vi "drive_calc.vi"(11 "Drive_inputs":T2) -> (3 "Drive_Outputs":T1)   [LabVIEW 2013]
uses:
  drive_inputs.ctl
  drive_outputs.ctl
panel:
  in  "Drive_Outputs 2":T1
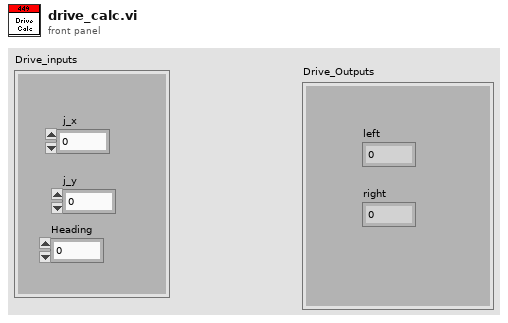
[diagram p1: front panel]
types:
  T1 = typedef "drive_outputs.ctl" = cluster{"left":dbl, "right":dbl}
  T2 = typedef "drive_inputs.ctl" = cluster{"j_x":dbl, "j_y":dbl, "Heading":dbl}
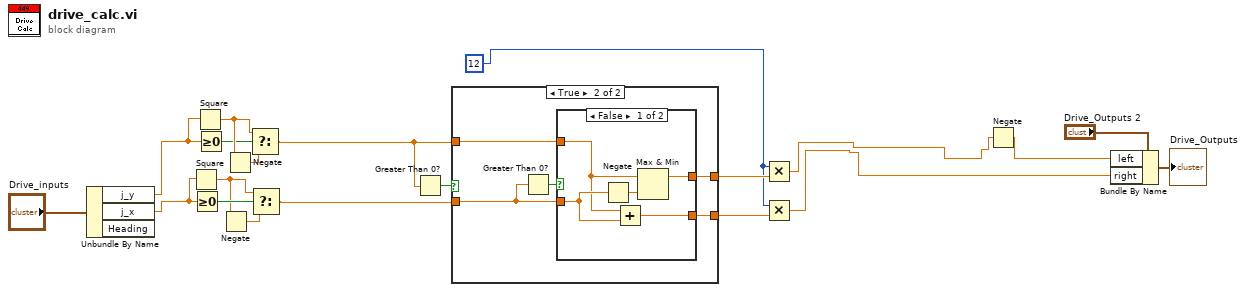
[diagram p0: block diagram]
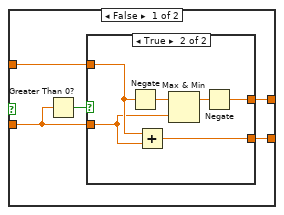
[diagram p2: hidden frame]
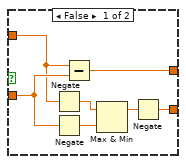
[diagram p3: hidden frame]
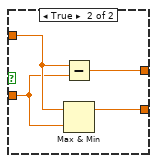
[diagram p4: hidden frame]
diagram:
  w13 = 12
  n1 = Unbundle By Name("Drive_inputs") -> ("j_y"=w4:dbl, "j_x"=w3:dbl)  [unwired: 1 out]
  n2 = Square(x=w3) -> (x^2=w11:dbl)
  n3 = Greater Or Equal To 0?(x=w3) -> (x >= 0?=w12:bool)
  n4 = Square(x=w4) -> (x^2=w8:dbl)
  n5 = Greater Or Equal To 0?(x=w4) -> (x >= 0?=w7:bool)
  n6 = Negate(x=w11) -> (-x=w10:dbl)
  n7 = Negate(x=w8) -> (-x=w9:dbl)
  n8 = Select(t=w8, s=w7, f=w9) -> (s? t:f=w6:dbl)
  n9 = Select(t=w11, s=w12, f=w10) -> (s? t:f=w5:dbl)
  n10 = Greater Than 0?(x=w6) -> (x > 0?=w17:bool)
  n11 = case shown="True" w17 {
    tunnel: w5 -> [w24 w42]
    tunnel: w6 -> [w23 w41]
    tunnel: [w22 w40] -> w16
    tunnel: [w21 w39] -> w15
    frame False {
      n12 = Greater Than 0?(x=w24) -> (x > 0?=w25:bool)
      n13 = case shown="True" w25 {
        tunnel: w24 -> [w32 w34]
        tunnel: w23 -> [w30 w35]
        tunnel: [w26 w36] -> w22
        tunnel: [w27 w33] -> w21
        frame False {
          n14 = Negate(x=w30) -> (-x=w31:dbl)
          n15 = Negate(x=w32) -> (-x=w29:dbl)
          n16 = Subtract(x=w30, y=w32) -> (x-y=w26:dbl)
          n17 = Max & Min(x=w31, y=w29) -> (max(x,y)=w28:dbl)  [unwired: 1 out]
          n18 = Negate(x=w28) -> (-x=w27:dbl)
        }
        frame True {
          n19 = Negate(x=w35) -> (-x=w38:dbl)
          n20 = Add(x=w35, y=w34) -> (x+y=w33:dbl)
          n21 = Max & Min(x=w38, y=w34) -> (max(x,y)=w37:dbl)  [unwired: 1 out]
          n22 = Negate(x=w37) -> (-x=w36:dbl)
        }
      }
    }
    frame True {
      n23 = Greater Than 0?(x=w42) -> (x > 0?=w43:bool)
      n24 = case shown="False" w43 {
        tunnel: w42 -> [w48 w50]
        tunnel: w41 -> [w45 w51]
        tunnel: [w46 w49] -> w40
        tunnel: [w44 w52] -> w39
        frame False {
          n25 = Negate(x=w48) -> (-x=w47:dbl)
          n26 = Add(x=w45, y=w48) -> (x+y=w44:dbl)
          n27 = Max & Min(x=w45, y=w47) -> (max(x,y)=w46:dbl)  [unwired: 1 out]
        }
        frame True {
          n28 = Subtract(x=w51, y=w50) -> (x-y=w49:dbl)
          n29 = Max & Min(x=w51, y=w50) -> (max(x,y)=w52:dbl)  [unwired: 1 out]
        }
      }
    }
  }
  n30 = Multiply(x=w13, y=w16) -> (x*y=w1:dbl)
  n31 = Multiply(x=w13, y=w15) -> (x*y=w14:dbl)
  n32 = Negate(x=w1) -> (-x=w2:dbl)
  n33 = Bundle By Name(cluster="Drive_Outputs 2", "left"=w2, "right"=w14) -> (→"Drive_Outputs":T1)
